vi "Get Printf Ref.vi"() -> (3 "Printf DVR":refnum<data-value>)   [LabVIEW 2013, in "SET_Printf.lvlib" / "LV_Printf Core.lvclass"]
uses:
  LV_Printf Core.lvclass
  Messages/General/LV_Printf Msg.lvclass
  LV_Printf Core.lvclass/LV_Printf Core.ctl
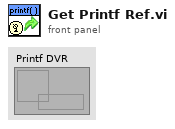
[diagram p1: front panel]
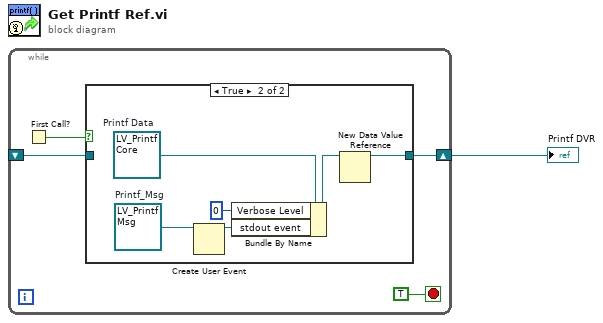
[diagram p0: block diagram]
diagram:
  n1 = while {
    shift-right: [w5] -> w1
    shift-left: _ -> [w2]
    stop <- TRUE stop-if-true
    n2 = First Call?() -> (First Call?: T/F=w4:bool)
    n3 = case shown="True" w4 {
      tunnel: [w6 w12] -> w5
      tunnel: w2 -> [w6 _]
      frame False {
      }
      frame True {
        w10 = refnum<class "LV_Printf Msg.lvclass"> refnum  # Printf_Msg
        w11 = refnum<class "LV_Printf Core.lvclass"> refnum  # Printf Data
        n4 = Create User Event(user event datatype=w10) -> (user event=w9:refnum<user-event>)  [unwired: 1 in, 1 out]
        n5 = Bundle By Name(cluster=w11, "Verbose Level"=0, "stdout event"=w9) -> (w8:refnum<class "LV_Printf Core.lvclass">)
        n6 = New Data Value Reference(data value=w8) -> (data value reference=w12:refnum<data-value>)  [unwired: 1 in, 1 out]
      }
    }
  }
  "Printf DVR" <- w1
